vi "Device Settings.vi"(8 "error in":errorcluster, 11 "objects in":T1) -> (0 "error out":errorcluster, 3 "objects out":T1)   [LabVIEW 2011]
uses:
  Controls/Class Objects.ctl
  Modules/File/Configuration/Configuration.lvclass
  Modules/Hardware/Power Supply/Power Supply.lvclass
  Modules/Hardware/Mass Flow Controller/Mass Flow Controller.lvclass
  Modules/Hardware/Detector/Detector.lvclass
  Modules/File/TDMS/TDMS.lvclass
  Functional Globals/Device Parameters.ctl
panel:
  in  "?":enum32{"Device Name", "Device Name 2"}(tab)
  in  "Device Name.Setpoint":dbl
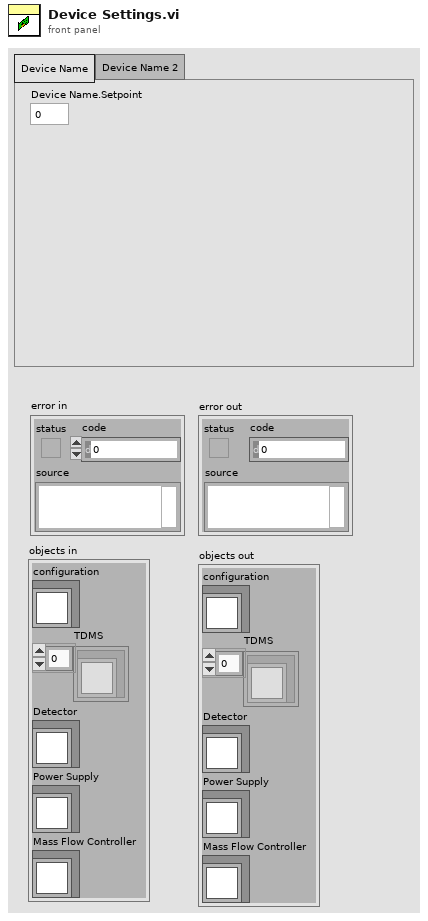
[diagram p1: front panel]
types:
  T1 = typedef "Class Objects.ctl" = cluster{"configuration":refnum<class "Configuration.lvclass">, "TDMS":refnum<class "TDMS.lvclass">[], "Power Supply":refnum<class "Power Supply.lvclass">, "Mass Flow Controller":refnum<class "Mass Flow Controller.lvclass">, "Detector":refnum<class "Detector.lvclass">}
  T2 = typedef "Device Parameters.ctl" = enum16{"Initialize", "Set Device Connections", "Set Device Settings", "Get Device Connections", "Get Device Settings"}
  T3 = typedef "Device Settings.ctl" = cluster{"Device Name":cluster{"Setpoint":dbl}}
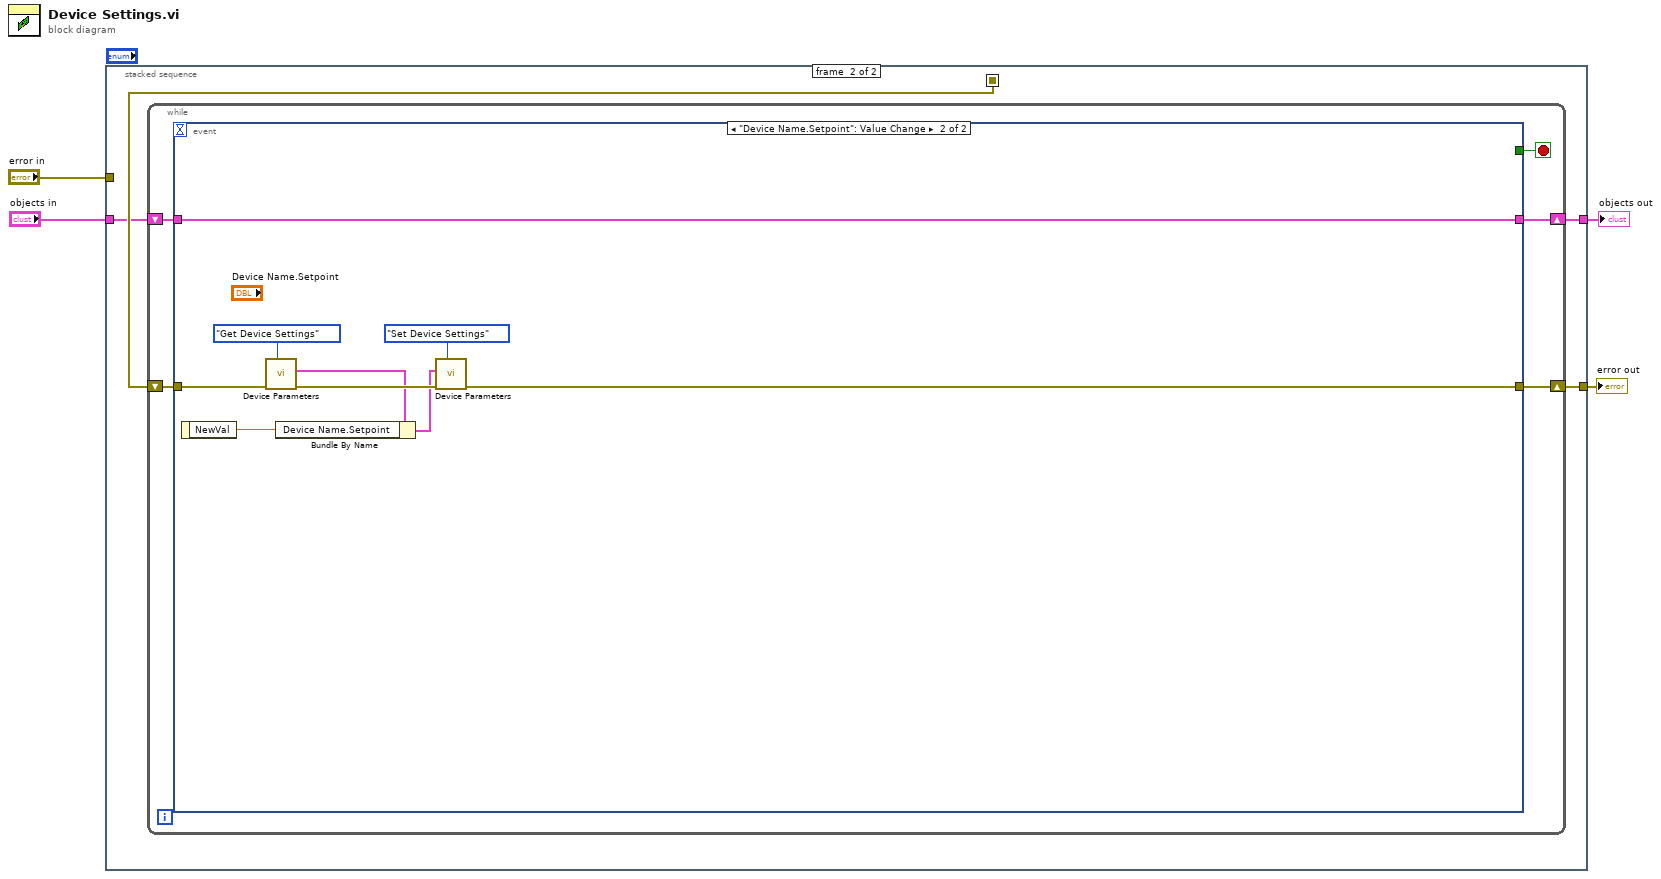
[diagram p0: block diagram]
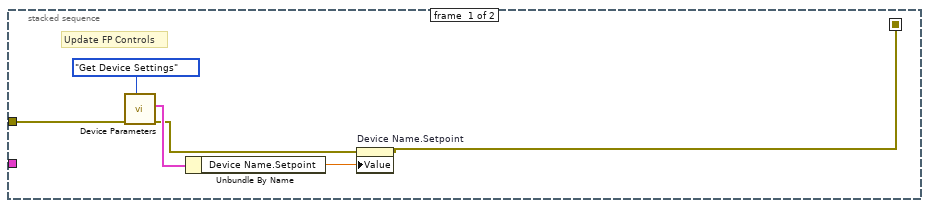
[diagram p2: hidden frame]
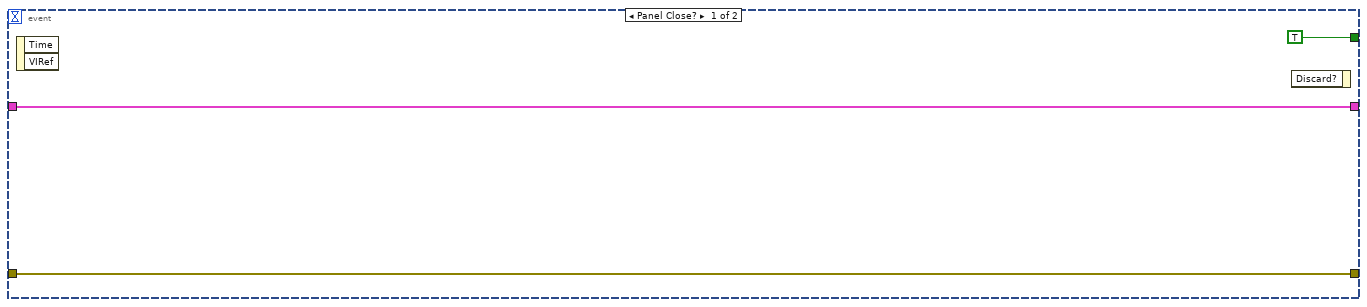
[diagram p3: hidden frame]
diagram:
  n1 = stacked-sequence {
    seq-local: [w5 _] -> [_ w14]
    tunnel: "error in" -> [w10 _]
    tunnel: [_ w11] -> w3
    tunnel: "objects in" -> [_ w13]
    tunnel: [_ w12] -> w1
    frame #0 {
      # "Update FP Controls"
      n2 = call "Device Parameters.vi"("command"=Device_Parameters."Get Device Settings", "error in"=w10) -> ("error out"=w6:errorcluster, "Device Settings OUT"=w8:T3)  [unwired: 7 in, 1 out]
      n3 = Unbundle By Name(w8) -> ("Device Name.Setpoint"=w7:dbl)
      n4 = property on="Device Name.Setpoint" class="DigNum (strict)"(error in=w6, "Value"=w7) -> (error out=w5:errorcluster)  [unwired: 1 in, 1 out]
    }
    frame #1 {
      n5 = while {
        shift-right: [w16] -> w12
        shift-left: w13 -> [w17]
        shift-right: [w15] -> w11
        shift-left: w14 -> [w19]
        stop <- w18 stop-if-true
        n6 = event shown="[1] \"Device Name.Setpoint\": Value Change" {
          selector: _ -> [_ _]
          dyn-events: _ -> [_ _]
          timeout: _ -> [_ _]
          tunnel: w19 -> [w22 w27]
          tunnel: [w22 w23] -> w15
          tunnel: [TRUE _] -> w18
          tunnel: w17 -> [w20 w31]
          tunnel: [w20 w31] -> w16
          event Panel Close? {
            n7 = event-data() -> ()  [unwired: 1 in, 2 out]
            n8 = event-data() -> ()  [unwired: 2 in, 1 out]
          }
          event "Device Name.Setpoint": Value Change {
            n9 = event-data() -> ("NewVal"=w25:dbl)  [unwired: 1 in]
            n10 = call "Device Parameters.vi"("command"=Device_Parameters."Get Device Settings", "error in"=w27) -> ("error out"=w28:errorcluster, "Device Settings OUT"=w26:T3)  [unwired: 7 in, 1 out]
            n11 = Bundle By Name(cluster=w26, "Device Name.Setpoint"=w25) -> (w24:T3)
            n12 = call "Device Parameters.vi"("command"=Device_Parameters."Set Device Settings", "error in"=w28, "Device Settings IN"=w24) -> ("error out"=w23:errorcluster)  [unwired: 6 in, 2 out]
          }
        }
      }
    }
  }
  "error out" <- w3
  "objects out" <- w1
